vi "cursor changer.vi"() -> ()   [LabVIEW 2020]
uses:
  <vilib>/Utility/cursorutil.llb/Set Cursor (Icon Pict).vi
panel:
  in  "icon":u16(ring)
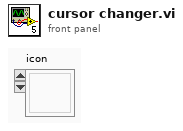
[diagram p1: front panel]
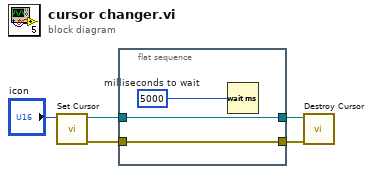
[diagram p0: block diagram]
diagram:
  n1 = call-poly <vilib>:"Set Cursor.vi"("icon"="icon") -> ("error out"=w3:errorcluster, "previous cursor ID"=w4:refnum<k1>)  [unwired: 9 in]
  n2 = flat-sequence {
    tunnel: w4 -> [w8]
    tunnel: w3 -> [w7]
    tunnel: [w8] -> w2
    tunnel: [w7] -> w1
    frame #0 {
      w6 = u32 5000  # milliseconds to wait
      n3 = Wait (ms)(milliseconds to wait=w6) -> ()  [unwired: 1 out]
    }
  }
  n4 = call <vilib>:"Destroy Cursor.vi"("cursor ID"=w2, "error in (no error)"=w1) -> ()  [unwired: 8 in, 1 out]
